vi "Counter.vi"() -> (3 "counts":i32)   [LabVIEW 2020]
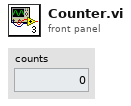
[diagram p1: front panel]
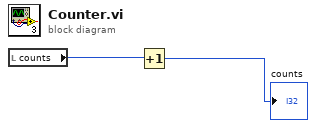
[diagram p0: block diagram]
diagram:
  n1 = local read "counts"() -> (w2:i32)
  n2 = Increment(x=w2) -> (x+1=→"counts":i32)
